vi "Get Year.vi"(10 "Day format":T1=enum."YY") -> (2 "Year":string)   [LabVIEW 2017]
uses:
  Typedefs/SN Components Enum.ctl
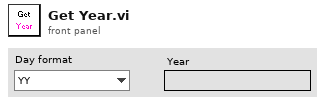
[diagram p1: front panel]
types:
  T1 = typedef "SN Components Enum.ctl" = enum16{"Constant String", "Incrementing number", "Space", "Day of the week (D)", "Day of the week (DD)", "Day of the month (D)", "Day of the month (DD)", "W", "WW", "MM", "YY", "YYYY"}
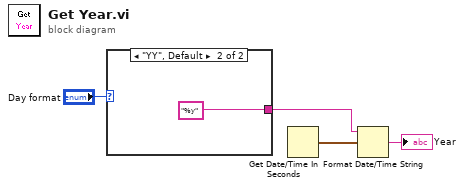
[diagram p0: block diagram]
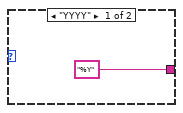
[diagram p2: hidden frame]
diagram:
  n1 = case shown="\"YY\", Default" "Day format" {
    tunnel: ["%Y" ("time format string (%c)") "%y" ("time format string (%c)")] -> w1
    frame "YYYY" {
    }
    frame "YY", Default {
    }
  }
  n2 = Get Date/Time In Seconds() -> (seconds since 1Jan1904=w4:timestamp)
  n3 = Format Date/Time String(time format string (%c)=w1, seconds (now)=w4) -> (date/time string=→"Year":string)  [unwired: 1 in]
